vi "Batch-Import-User-Channels Main Page.vi"(8 "error in (no error)":errorcluster, 11 "Node Ptr":T1 format="%.0x") -> (0 "error out":errorcluster)   [LabVIEW 2015, in "Batch-Import-User-Channels Custom Device.lvlib"]
uses:
  Batch-Import-User-Channels Custom Device.lvlib
  <vilib>/NI Veristand/Custom Device API/Custom Device Item Ref.ctl
  <vilib>/NI Veristand/Custom Device API/Custom Device Channel.ctl
  <vilib>/NI Veristand/Custom Device API/Custom Device Channel Type.ctl
  <vilib>/NI Veristand/Custom Device API/Custom Device API.lvlib
panel:
  in  "Add Button":bool
  in  "Header":cluster{"Section Name":string}={"Section Name"="Custom Device Item Settings"}
  in  "Description":string
  in  "Name":string
  # "BICU-Channels对应Channel Folder\nBICU-Channel 0...对应Channel Name\n数值直接对应初始值\n字符串值对应的规则是:初始值@通道描述"
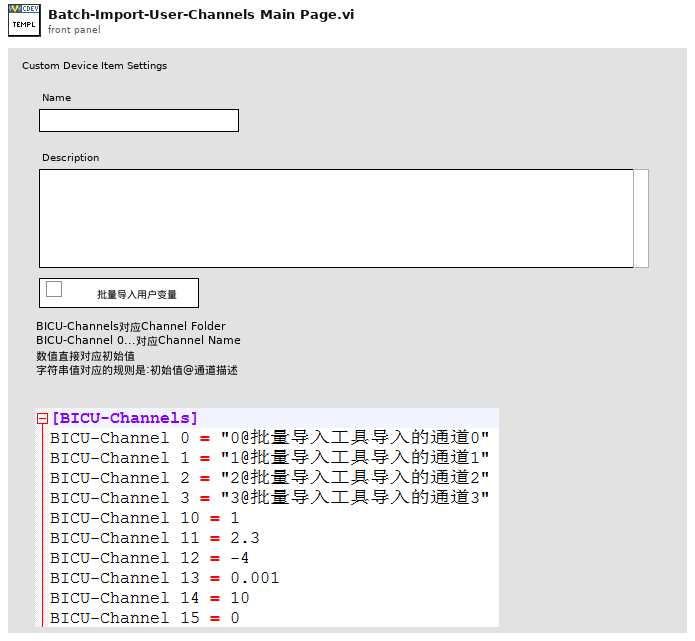
[diagram p1: front panel]
types:
  T1 = typedef "Custom Device API.lvlib/Custom Device Item Ref.ctl" = u64
  T2 = typedef "Custom Device API.lvlib/Custom Device Item Info.ctl" = cluster{"Name":string, "Is Channel":bool, "GUID":string, "Is Waveform":bool}
  T3 = typedef "Custom Device API.lvlib/Custom Device Channel.ctl" = cluster{"Type":T4, "Units":string, "Default Value":dbl, "Faultable":bool, "Scalable":bool}
  T4 = typedef "Custom Device API.lvlib/Custom Device Channel Type.ctl" = enum16{"Input", "Output"}
  T5 = typedef "Custom Device API.lvlib/Custom Device Commands.ctl" = enum16{"Default", "Item renamed", "Shutdown", "Dynamic button pressed"}
  T6 = cluster{"Group":string, "Channels":cluster{"Name":string, "DefaultValue":dbl, "Desp":string}[]}[]
  T7 = cluster{"Name":string, "DefaultValue":dbl, "Desp":string}[]
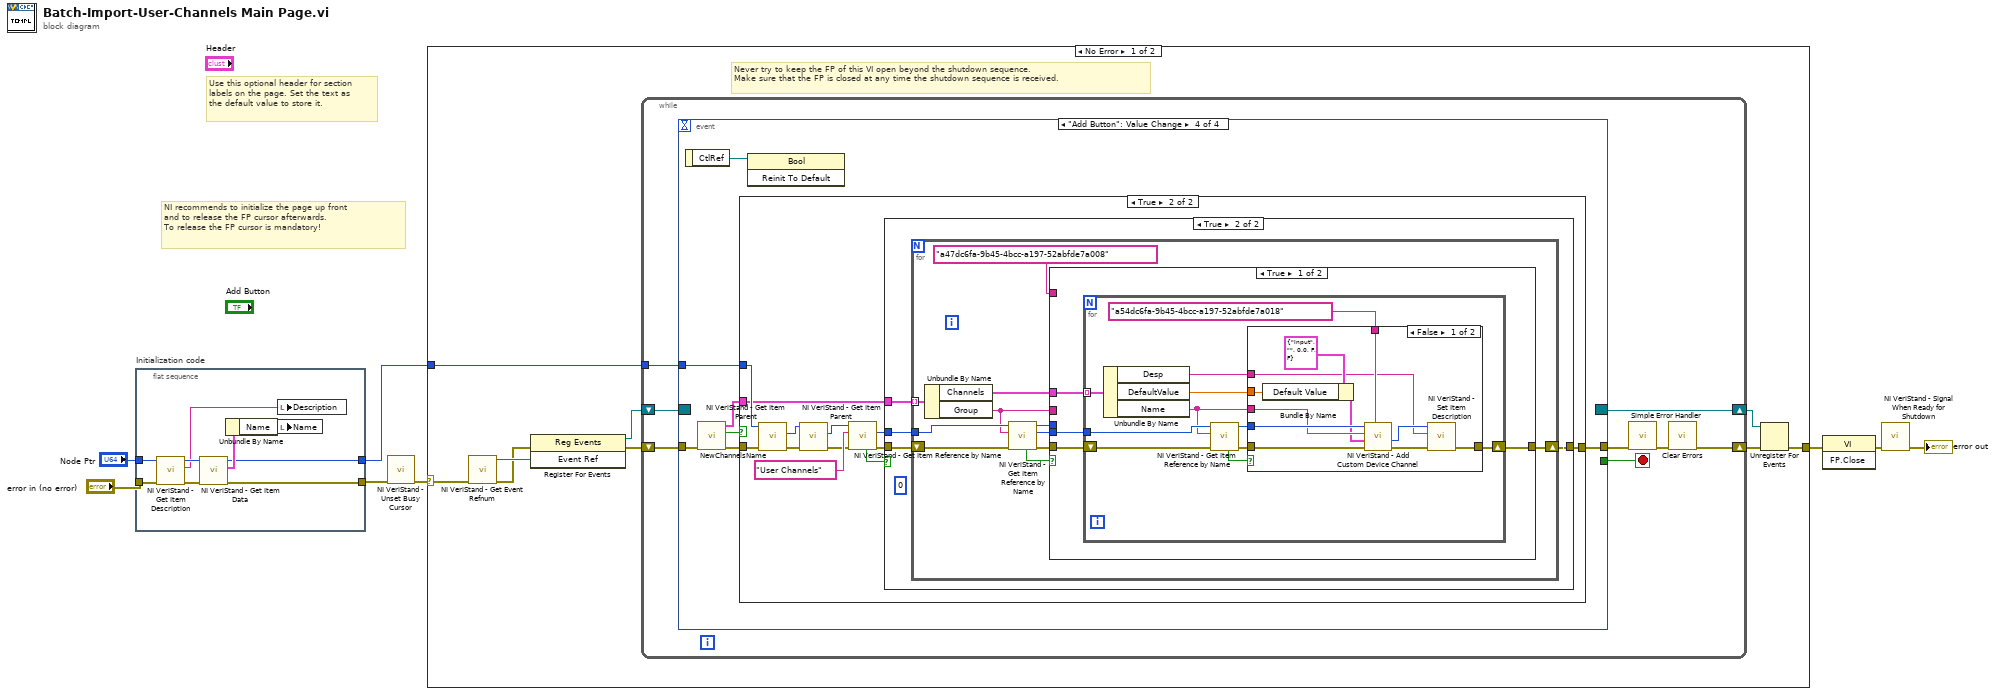
[diagram p0: block diagram]
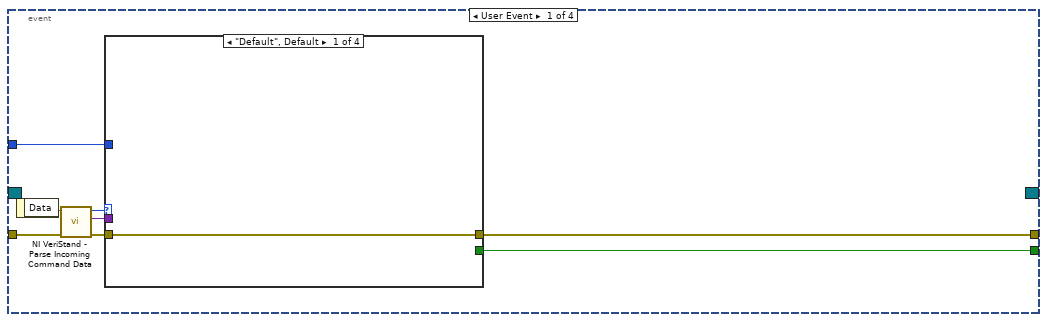
[diagram p2: hidden frame]
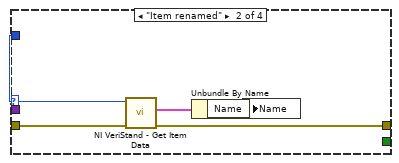
[diagram p3: hidden frame]
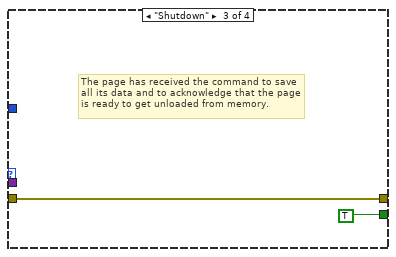
[diagram p4: hidden frame]
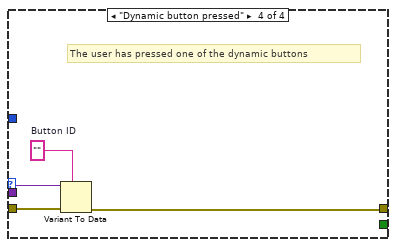
[diagram p5: hidden frame]
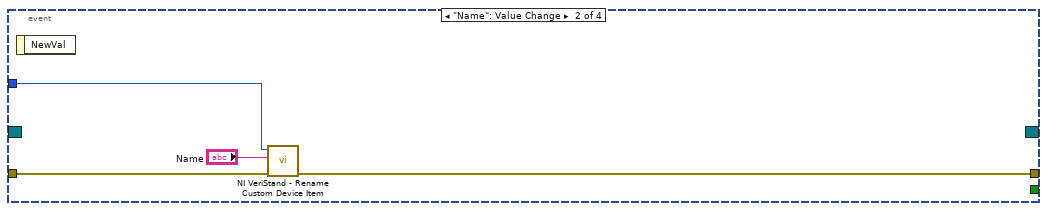
[diagram p6: hidden frame]
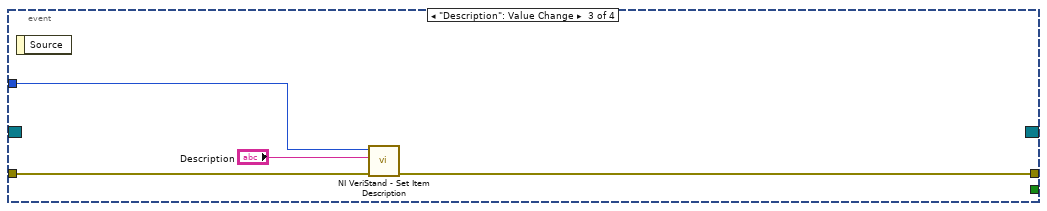
[diagram p7: hidden frame]
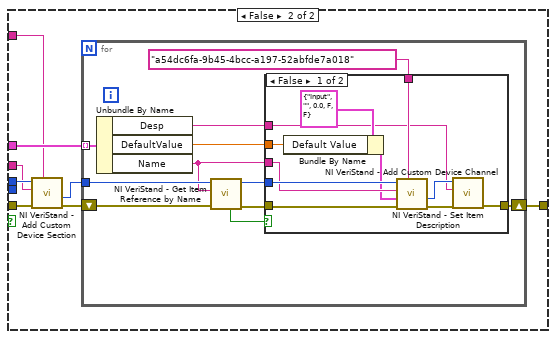
[diagram p11: hidden frame]
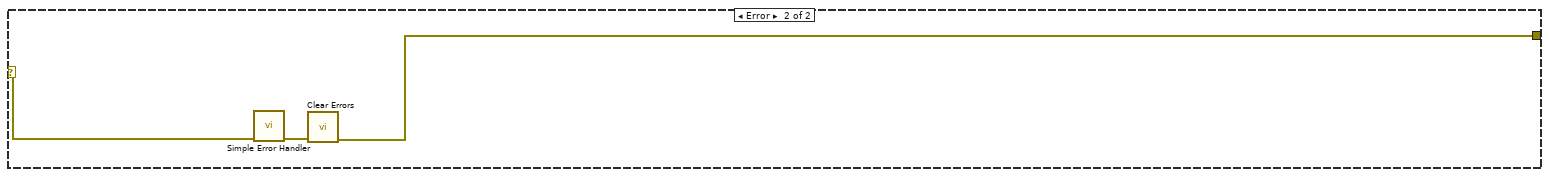
[diagram p13: hidden frame]
diagram:
  # "Use this optional header for section labels on the page. Set the text as the default value to store it."
  # "NI recommends to initialize the page up front\nand to release the FP cursor afterwards.\nTo release the FP cursor is mandatory!"
  n1 = flat-sequence "Initialization code" {
    tunnel: "error in (no error)" -> [w16]
    tunnel: "Node Ptr" -> [w15]
    tunnel: [w10] -> w4
    tunnel: [w9] -> w1
    frame #0 {
      n2 = call <vilib>:"NI VeriStand - Get Item Description.vi"("error in (no error)"=w16, "Item Ref in"=w15) -> ("error out"=w13:errorcluster, "Description"=w14:string, "Item Ref out"=w17:T1)  [unwired: 7 out]
      n3 = call <vilib>:"NI VeriStand - Get Item Data.vi"("error in (no error)"=w13, "Item Ref in"=w17) -> ("error out"=w10:errorcluster, "Item Info"=w12:T2, "Item Ref out"=w9:T1)  [unwired: 7 out]
      n4 = Unbundle By Name(w12) -> ("Name"=w11:string)
      n5 = local write "Description"(w14) -> ()
      n6 = local write "Name"(w11) -> ()
    }
  }
  n7 = call <vilib>:"NI VeriStand - Unset Busy Cursor.vi"("error in (no error)"=w4) -> ("error out"=w3:errorcluster)  [unwired: 10 out]
  n8 = case shown="No Error" w3 {
    selector: w3 -> [w19 w159]
    tunnel: [w24 w157] -> w8
    tunnel: w1 -> [w20 _]
    frame No Error {
      # "Never try to keep the FP of this VI open beyond the shutdown sequence.\nMake sure that the FP is closed at any time the shutdown sequence is received."
      n9 = call <vilib>:"NI VeriStand - Get Event Refnum.vi"("error in (no error)"=w19) -> ("error out"=w18:errorcluster, "Event Ref"=w23:refnum<user-event>)  [unwired: 9 out]
      n10 = register-events(error in=w18, w23) -> (reference out=w21:refnum<event-registration>, error out=w22:errorcluster)  [unwired: 1 in]
      n11 = while {
        tunnel: w20 -> [w30]
        shift-right: [w27] -> w25
        shift-left: w22 -> [w33]
        shift-right: [w34] -> w26
        shift-left: w21 -> [w32]
        stop <- w31 stop-if-true
        n12 = event shown="[3] \"Add Button\": Value Change" {
          selector: w32 -> [_ _ _ _]
          dyn-events: [_ _ _ _] -> w34
          timeout: _ -> [_ _ _ _]
          tunnel: w33 -> [w42 w58 w61 w67]
          tunnel: [w38 _ _ _] -> w31
          tunnel: [w37 w57 w60 w68] -> w29
          tunnel: w30 -> [w36 w56 w62 w69]
          event User Event {
            n13 = event-data() -> ("Data"=w41:string)  [unwired: 1 out]
            n14 = call <vilib>:"NI VeriStand - Parse Incoming Command Data.vi"("error in (no error)"=w42, "Incoming data"=w41) -> ("error out"=w40:errorcluster, "Outgoing data"=w35:variant, "Action"=w39:T5)  [unwired: 7 out]
            n15 = case shown="\"Default\", Default" w39 {
              tunnel: w40 -> [w43 w48 w49 w54]
              tunnel: [_ _ TRUE _] -> w38
              tunnel: [w43 w45 w49 w51] -> w37
              tunnel: w36 -> [_ w47 _ _]
              tunnel: w35 -> [_ _ _ w53]
              frame "Default", Default {
              }
              frame "Item renamed" {
                n16 = call <vilib>:"NI VeriStand - Get Item Data.vi"("error in (no error)"=w48, "Item Ref in"=w47) -> ("error out"=w45:errorcluster, "Item Info"=w46:T2)  [unwired: 8 out]
                n17 = Unbundle By Name(w46) -> ("Name"=w44:string)
                n18 = local write "Name"(w44) -> ()
              }
              frame "Shutdown" {
                # "The page has received the command to save all its data and to acknowledge that the page is ready to get unloaded from memory."
              }
              frame "Dynamic button pressed" {
                w52 = ""  # Button ID
                # "The user has pressed one of the dynamic buttons"
                n19 = Variant To Data(error in=w54, type=w52, Variant=w53) -> (error out=w51:errorcluster)  [unwired: 1 out]
              }
            }
          }
          event "Name": Value Change {
            n20 = event-data() -> ()  [unwired: 2 out]
            n21 = call <vilib>:"NI VeriStand - Rename Custom Device Item.vi"("error in (no error)"=w58, "New Name"="Name", "Item Ref in"=w56) -> ("error out"=w57:errorcluster)  [unwired: 1 in, 7 out]
          }
          event "Description": Value Change {
            n22 = event-data() -> ()  [unwired: 2 out]
            n23 = call <vilib>:"NI VeriStand - Set Item Description.vi"("error in (no error)"=w61, "Description"="Description", "Item Ref in"=w62) -> ("error out"=w60:errorcluster)  [unwired: 8 out]
          }
          event "Add Button": Value Change {
            n24 = event-data() -> ("CtlRef"=w64:refnum<vi>)  [unwired: 1 out]
            n25 = call "NewChannelsName.vi"("error in (no error)"=w67) -> ("error out"=w66:errorcluster, "Confirm"=w65:bool, "AutoChls"=w63:T6)  [unwired: 7 in, 1 out]
            n26 = case shown="True" w65 {
              tunnel: w69 -> [_ w79]
              tunnel: [w70 w78] -> w68
              tunnel: w66 -> [w70 w73]
              tunnel: w63 -> [_ w71]
              frame False {
              }
              frame True {
                n27 = call <vilib>:"NI VeriStand - Get Item Parent.vi"("error in (no error)"=w73, "Item Ref in"=w79) -> ("error out"=w77:errorcluster, "Parent Ref"=w76:T1)  [unwired: 6 in, 2 out]
                n28 = call <vilib>:"NI VeriStand - Get Item Parent.vi"("error in (no error)"=w77, "Item Ref in"=w76) -> ("error out"=w74:errorcluster, "Parent Ref"=w75:T1)  [unwired: 6 in, 2 out]
                n29 = call <vilib>:"NI VeriStand - Get Item Reference by Name.vi"("error in (no error)"=w74, "Item Name"="User Channels", "Parent Ref in"=w75) -> ("error out"=w81:errorcluster, "Item Ref"=w82:T1, "Found"=w72:bool)  [unwired: 5 in, 1 out]
                n30 = case shown="True" w72 {
                  tunnel: w82 -> [_ w85]
                  tunnel: w81 -> [w83 w86]
                  tunnel: [w83 w87] -> w78
                  tunnel: w71 -> [_ w84]
                  frame False {
                  }
                  frame True {
                    (unwired) 0 ("Slide")
                    n31 = for {
                      tunnel: w85 -> [w96]
                      shift-right: [w98] -> w87
                      shift-left: w86 -> [w97]
                      tunnel: w84 -> [w91] mode=indexing
                      n32 = Unbundle By Name(w91) -> ("Channels"=w89:T7, "Group"=w90:string)
                      n33 = call <vilib>:"NI VeriStand - Get Item Reference by Name.vi"("error in (no error)"=w97, "Item Name"=w90, "Parent Ref in"=w96) -> ("error out"=w94:errorcluster, "Item Ref"=w93:T1, "Parent Ref out"=w92:T1, "Found"=w95:bool)  [unwired: 5 in]
                      n34 = case shown="True" w95 {
                        tunnel: [w102 w133] -> w98
                        tunnel: w89 -> [w101 w132]
                        tunnel: w94 -> [w99 w129]
                        tunnel: w93 -> [w100 _]
                        tunnel: w92 -> [_ w131]
                        tunnel: w90 -> [_ w130]
                        tunnel: "a47dc6fa-9b45-4bcc-a197-52abfde7a008" -> [_ w126]
                        frame True {
                          n35 = for {
                            tunnel: w100 -> [w111]
                            shift-right: [w113] -> w102
                            shift-left: w99 -> [w112]
                            tunnel: w101 -> [w106] mode=indexing
                            n36 = Unbundle By Name(w106) -> ("Desp"=w103:string, "DefaultValue"=w104:dbl, "Name"=w105:string)
                            n37 = call <vilib>:"NI VeriStand - Get Item Reference by Name.vi"("error in (no error)"=w112, "Item Name"=w105, "Parent Ref in"=w111) -> ("error out"=w109:errorcluster, "Parent Ref out"=w108:T1, "Found"=w110:bool)  [unwired: 5 in, 1 out]
                            n38 = case shown="False" w110 {
                              tunnel: [w116 w125] -> w113
                              tunnel: w109 -> [w123 w125]
                              tunnel: w108 -> [w124 _]
                              tunnel: w105 -> [w121 _]
                              tunnel: "a54dc6fa-9b45-4bcc-a197-52abfde7a018" -> [w120 _]
                              tunnel: w104 -> [w118 _]
                              tunnel: w103 -> [w114 _]
                              frame False {
                                n39 = Bundle By Name(cluster=T3 {"Type"=enum."Input", "Units"="", "Default Value"=0.0, "Faultable"=FALSE, "Scalable"=FALSE} ("Channel"), "Default Value"=w118) -> (w119:T3)
                                n40 = call <vilib>:"NI VeriStand - Add Custom Device Channel.vi"("GUID (Default Channel)"=w120, "error in (no error)"=w123, "Channel"=w119, "Channel Name"=w121, "Parent Ref in"=w124) -> ("error out"=w117:errorcluster, "Channel Ref"=w115:T1)  [unwired: 3 in, 2 out]
                                n41 = call <vilib>:"NI VeriStand - Set Item Description.vi"("error in (no error)"=w117, "Description"=w114, "Item Ref in"=w115) -> ("error out"=w116:errorcluster)  [unwired: 6 in, 2 out]
                              }
                              frame True {
                              }
                            }
                          }
                        }
                        frame False {
                          n42 = call <vilib>:"NI VeriStand - Add Custom Device Section.vi"("GUID (Default Section)"=w126, "error in (no error)"=w129, "Section Name"=w130, "Parent Ref in"=w131) -> ("error out"=w128:errorcluster, "Section Ptr"=w127:T1)  [unwired: 4 in, 2 out]
                          n43 = for {
                            tunnel: w127 -> [w142]
                            shift-right: [w144] -> w133
                            shift-left: w128 -> [w143]
                            tunnel: w132 -> [w137] mode=indexing
                            n44 = Unbundle By Name(w137) -> ("Desp"=w134:string, "DefaultValue"=w135:dbl, "Name"=w136:string)
                            n45 = call <vilib>:"NI VeriStand - Get Item Reference by Name.vi"("error in (no error)"=w143, "Item Name"=w136, "Parent Ref in"=w142) -> ("error out"=w140:errorcluster, "Parent Ref out"=w139:T1, "Found"=w141:bool)  [unwired: 5 in, 1 out]
                            n46 = case shown="False" w141 {
                              tunnel: [w145 w156] -> w144
                              tunnel: w140 -> [w154 w156]
                              tunnel: w139 -> [w155 _]
                              tunnel: w136 -> [w152 _]
                              tunnel: "a54dc6fa-9b45-4bcc-a197-52abfde7a018" -> [w151 _]
                              tunnel: w135 -> [w149 _]
                              tunnel: w134 -> [w147 _]
                              frame False {
                                n47 = Bundle By Name(cluster=T3 {"Type"=enum."Input", "Units"="", "Default Value"=0.0, "Faultable"=FALSE, "Scalable"=FALSE} ("Channel"), "Default Value"=w149) -> (w150:T3)
                                n48 = call <vilib>:"NI VeriStand - Add Custom Device Channel.vi"("GUID (Default Channel)"=w151, "error in (no error)"=w154, "Channel"=w150, "Channel Name"=w152, "Parent Ref in"=w155) -> ("error out"=w146:errorcluster, "Channel Ref"=w148:T1)  [unwired: 3 in, 2 out]
                                n49 = call <vilib>:"NI VeriStand - Set Item Description.vi"("error in (no error)"=w146, "Description"=w147, "Item Ref in"=w148) -> ("error out"=w145:errorcluster)  [unwired: 6 in, 2 out]
                              }
                              frame True {
                              }
                            }
                          }
                        }
                      }
                    }
                  }
                }
              }
            }
            n50 = invoke class="Bool" method="Reinit To Default"(reference=w64) -> ()  [unwired: 2 in, 3 out]
          }
        }
        n51 = call <vilib>:"Simple Error Handler.vi"("error in (no error)"=w29) -> ("error out"=w28:errorcluster)  [unwired: 1 in, 7 out]
        n52 = call <vilib>:"Clear Errors.vi"("error in (no error)"=w28) -> ("error out"=w27:errorcluster)  [unwired: 1 in, 5 out]
      }
      n53 = Unregister For Events(event registration refnum=w26, error in=w25) -> (error out=w24:errorcluster)
    }
    frame Error {
      n54 = call <vilib>:"Simple Error Handler.vi"("error in (no error)"=w159) -> ("error out"=w158:errorcluster)  [unwired: 1 in, 7 out]
      n55 = call <vilib>:"Clear Errors.vi"("error in (no error)"=w158) -> ("error out"=w157:errorcluster)  [unwired: 1 in, 5 out]
    }
  }
  n56 = invoke class="VI" method="FP.Close"(error in=w8) -> (error out=w7:errorcluster)  [unwired: 2 in, 2 out]
  n57 = call <vilib>:"NI VeriStand - Signal When Ready for Shutdown.vi"("error in (no error)"=w7) -> ("error out"=→"error out":errorcluster)  [unwired: 10 out]
